vi "Frame array-Build.vi"(0 "Single-frame buffer (in)":dbl[](array[numeric]), 1 "Logging queue element":T1={"Imaging Protocol"=enum."Live Imaging", "Number of Trials"=0, "Frame Size"=512, "# Averaged frames"=0, "Dwell time (us)"=0.0, "Index of Z-plane"=0, "Timelapse?"=FALSE, "Logging process is active"=FALSE, "Speed logging enabled"=FALSE, "tdms file ref"=refnum, "path"=path "", "Trial Number"=0, "Expected # points acquired"=FALSE, "Manually stopped"=FALSE, "Last trial"=FALSE, "Ch0 data"=[], "Ch1 data"=[], "Image Time"=[], "Continuous Time"=[], "Points acquired"={"Ch0 last trial"=0, "Ch1 last trial"=0, "All trials"=0}, "HW Timings File"=refnum} {"Frame Size" items=["100X100"=100, "128X128"=128, "200X200"=200, "256X256"=256, "512X512"=512, "1024x1024"=1024, "2048x2048"=2048]; "Dwell time (us)" format="%#.6g"}, 5 "New chunk of scaled data (single channel)":dbl[](array[numeric]), 9 "Number of points in single-frame buffer (in)":i32, 11 "Frame values sum (in)":dbl[](array[numeric]), 12 "Averaged frames count (in)":i32, 13 "Number of channels in input data array":i32=1) -> (3 "Frame Data":dbl[](array[numeric]), 4 "Single-frame buffer (out)":dbl[](array[numeric]), 6 "Frame completed/generate image":bool, 10 "Number of points in single-frame buffer (out)":i32, 14 "Averaged frames count (out)":i32, 15 "Frame values sum (out)":dbl[](array[numeric]))   [LabVIEW 2017]
uses:
  Typedefs/Logging queue element.ctl
  Typedefs/Imaging Protocols enum.ctl
  Typedefs/Frame Size.ctl
  Typedefs/Acquired points count.ctl
panel:
  out "# Averaged frames":u16
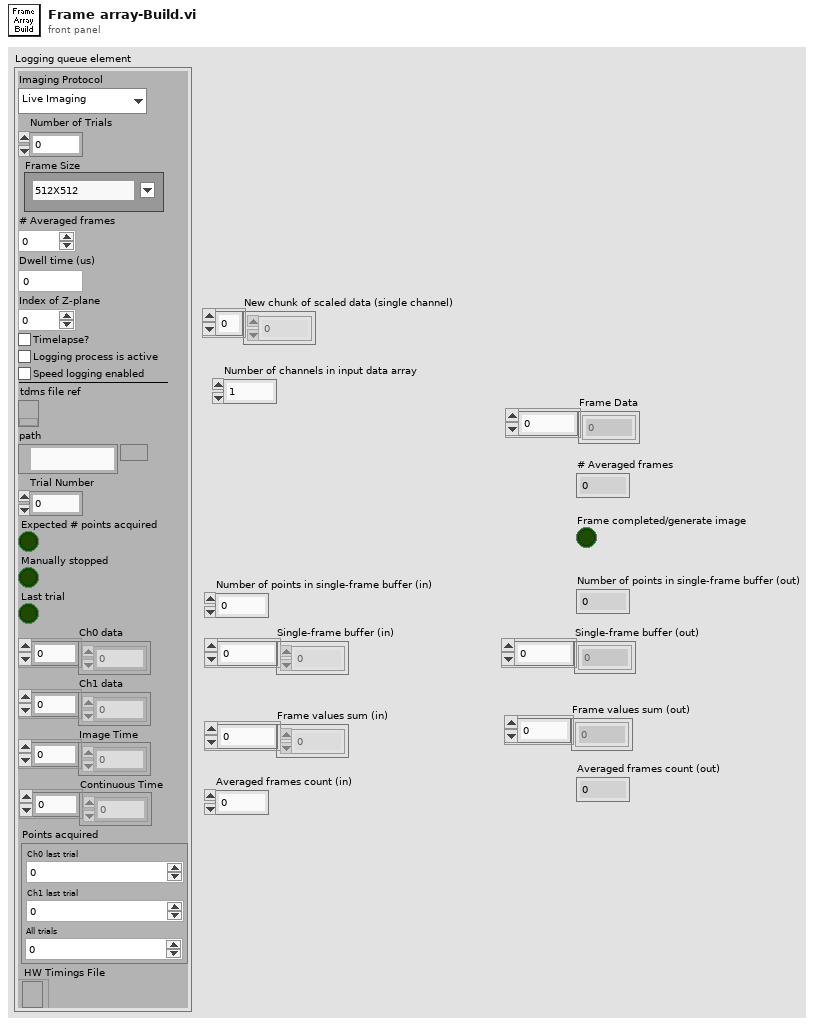
[diagram p1: front panel]
types:
  T1 = typedef "Logging queue element.ctl" = cluster{"Imaging Protocol":T2, "Number of Trials":u16, "Frame Size":T3, "# Averaged frames":u16, "Dwell time (us)":dbl, "Index of Z-plane":i32, "Timelapse?":bool, "Logging process is active":bool, "Speed logging enabled":bool, "tdms file ref":refnum<k34>, "path":path, "Trial Number":i32, "Expected # points acquired":bool, "Manually stopped":bool, "Last trial":bool, "Ch0 data":u32[], "Ch1 data":u32[], "Image Time":u64[], "Continuous Time":u64[], "Points acquired":T4, "HW Timings File":refnum<file>}
  T2 = typedef "Imaging Protocols enum.ctl" = enum16{"AOL Z-Stack", "Motor Z Stack", "Functional Acquisition", "Single Plane Acquisition", "Volume Acquisition", "Live Imaging", "Live Plane Imaging", "Live Volume Imaging"}
  T3 = typedef "Frame Size.ctl" = u16
  T4 = typedef "Acquired points count.ctl" = cluster{"Ch0 last trial":u64, "Ch1 last trial":u64, "All trials":u64}
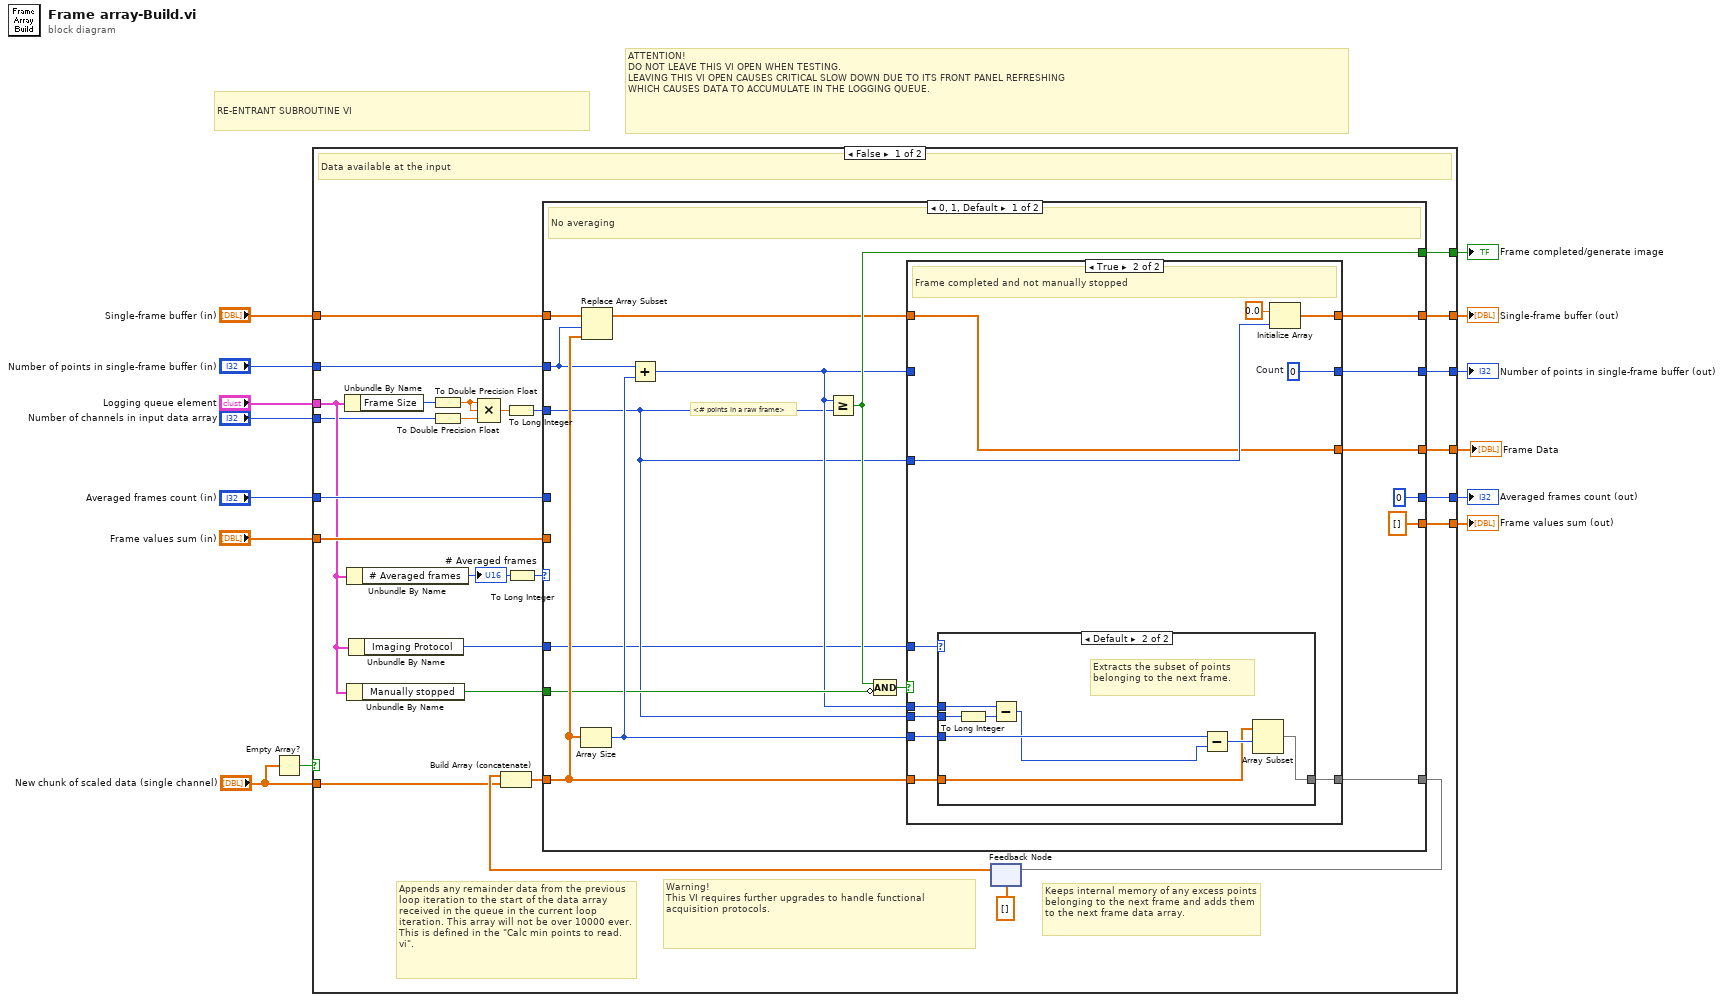
[diagram p0: block diagram]
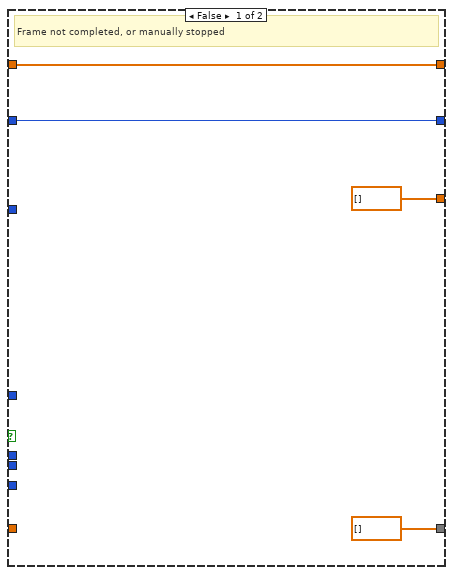
[diagram p2: hidden frame]
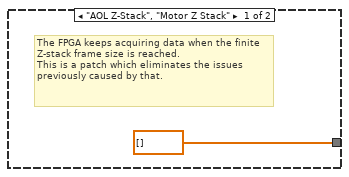
[diagram p3: hidden frame]
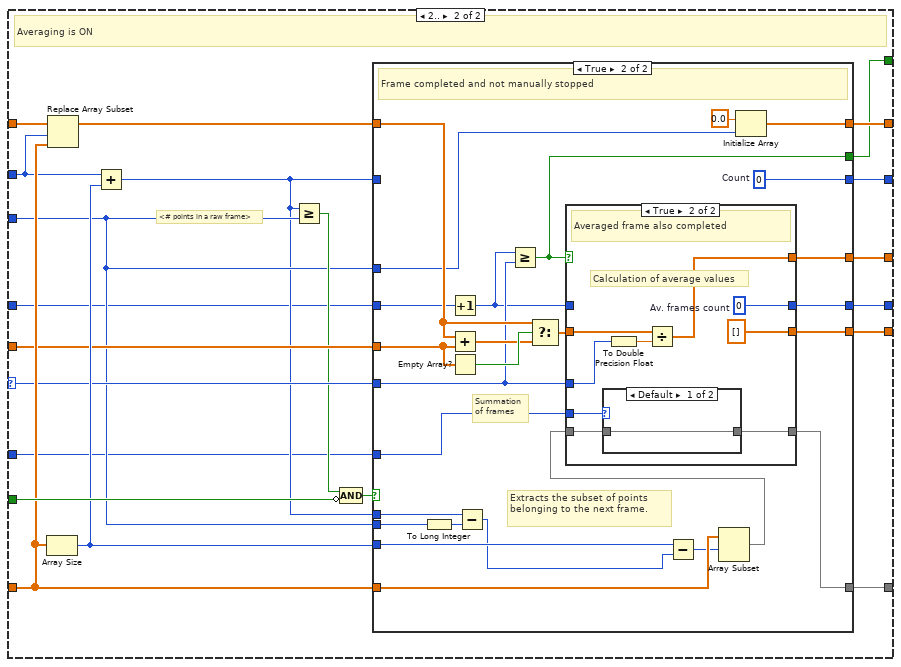
[diagram p4: hidden frame]
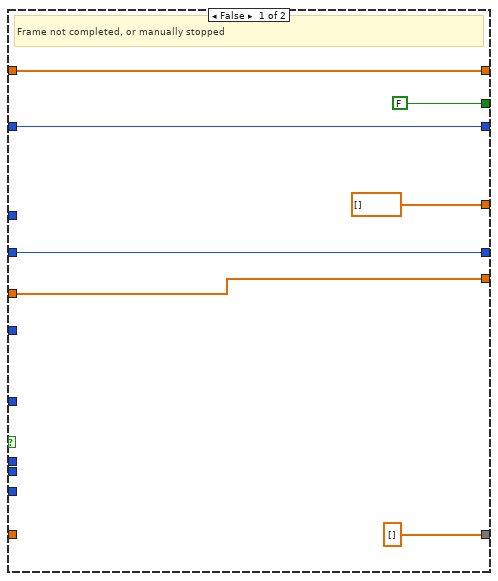
[diagram p5: hidden frame]
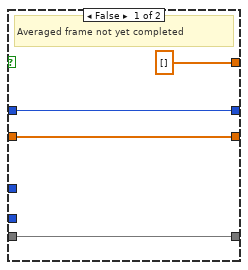
[diagram p6: hidden frame]
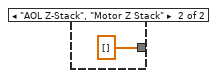
[diagram p7: hidden frame]
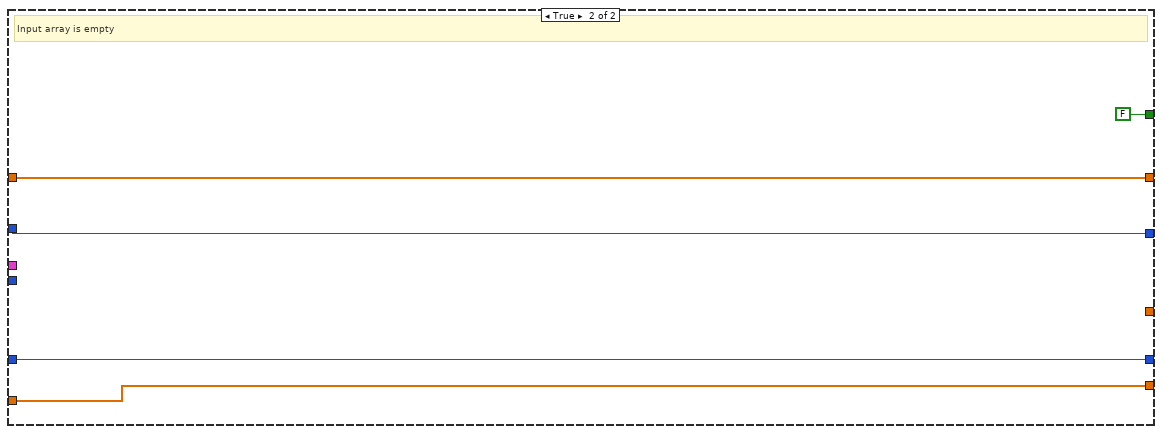
[diagram p8: hidden frame]
diagram:
  # "ATTENTION!\nDO NOT LEAVE THIS VI OPEN WHEN TESTING.\nLEAVING THIS VI OPEN CAUSES CRITICAL SLOW DOWN DUE TO ITS FRONT PANEL REFRESHING\nWHICH CAUSES DATA TO ACCUMULATE IN THE LOGGING QUEUE."
  # "RE-ENTRANT SUBROUTINE VI"
  n1 = Empty Array?(array="New chunk of scaled data (single channel)") -> (empty?=w1:bool)
  n2 = case shown="False" w1 {
    tunnel: "Number of points in single-frame buffer (in)" -> [w40 w154]
    tunnel: [w39 FALSE] -> w13
    tunnel: "Single-frame buffer (in)" -> [w38 w155]
    tunnel: [w37 w154] -> w11
    tunnel: "Frame values sum (in)" -> [w36 w151]
    tunnel: [w35 w151] -> w9
    tunnel: [w34 w155] -> w8
    tunnel: [w33 _] -> w7
    tunnel: [w32 w153] -> w6
    tunnel: "Averaged frames count (in)" -> [w31 w153]
    tunnel: "Logging queue element" -> [w20 _]
    tunnel: "New chunk of scaled data (single channel)" -> [w18 _]
    tunnel: "Number of channels in input data array" -> [w17 _]
    frame False {
      # "Warning!\nThis VI requires further upgrades to handle functional acquisition protocols."
      # "Appends any remainder data from the previous loop iteration to the start of the data array received in the queue in the current loop iteration. This array will not be over 10000 ever. This is defined in the \"Calc min points to read.vi\"."
      # "Keeps internal memory of any excess points belonging to the next frame and adds them to the next frame data array."
      # "Data available at the input"
      n3 = Unbundle By Name(w20) -> ("Frame Size"=w29:T3)
      n4 = Unbundle By Name(w20) -> ("# Averaged frames"=w24:u16)
      "# Averaged frames" <- w24
      n5 = Unbundle By Name(w20) -> ("Manually stopped"=w27:bool)
      n6 = Unbundle By Name(w20) -> ("Imaging Protocol"=w19:T2)
      n7 = To Double Precision Float(number=w29) -> (double precision float=w26:dbl)
      n8 = To Double Precision Float(number=w17) -> (double precision float=w16:dbl)
      n9 = Compound Arithmetic op=MULTIPLY(w26, w26, w16) -> (w25:dbl)
      n10 = To Long Integer(number=w25) -> (32bit integer=w15:i32)
      n11 = To Long Integer(number=w24) -> (32bit integer=w22:i32)
      n12 = feedback #1(dbl[] []) -> (w23:dbl[])
      n13 = Build Array (concatenate)(w23, w18) -> (w21:dbl[])
      n14 = case shown="0, 1, Default" w22 {
        selector: w22 -> [_ w94]
        tunnel: [w57 w102] -> w30
        tunnel: [w56 w84] -> w39
        tunnel: w27 -> [w49 w100]
        tunnel: w21 -> [w54 w99]
        tunnel: [w47 w89] -> w34
        tunnel: w38 -> [w53 w98]
        tunnel: w40 -> [w52 w97]
        tunnel: w15 -> [w45 w91]
        tunnel: [w46 w87] -> w37
        tunnel: w36 -> [_ w95]
        tunnel: [dbl[] [] ("Averaged frame values sum (in)") w92] -> w35
        tunnel: [w44 w86] -> w33
        tunnel: [0 ("Av. frames count") w85] -> w32
        tunnel: w31 -> [_ w83]
        tunnel: w19 -> [w41 w82]
        frame 0, 1, Default {
          # "<# points in a raw frame>"
          # "No averaging"
          n15 = Array Size(array=w54) -> (size(s)=w51:i32)
          n16 = Replace Array Subset "Replace Array Subset"(array=w53, new element=w54, index=w52) -> (w42:dbl[])
          n17 = Add(x=w52, y=w51) -> (x+y=w48:i32)
          n18 = Greater Or Equal?(x=w48, y=w45) -> (x >= y?=w56:bool)
          n19 = Compound Arithmetic op=AND(w56, invert w49) -> (w55:bool)
          n20 = case shown="True" w55 {
            tunnel: w48 -> [_ w72]
            tunnel: w54 -> [_ w70]
            tunnel: w51 -> [_ w71]
            tunnel: [dbl[] [] w69] -> w57
            tunnel: w45 -> [_ w68]
            tunnel: w42 -> [w59 w63]
            tunnel: w48 -> [w60 _]
            tunnel: [w60 w64] -> w46
            tunnel: [w59 w66] -> w47
            tunnel: w45 -> [_ w65]
            tunnel: [dbl[] [] w63] -> w44
            tunnel: w41 -> [_ w62]
            frame False {
              # "Frame not completed, or manually stopped"
            }
            frame True {
              w64 = 0  # Count
              # "Frame completed and not manually stopped"
              n21 = case shown="Default" w62 {
                tunnel: w72 -> [_ w81]
                tunnel: w71 -> [_ w79]
                tunnel: w70 -> [_ w76]
                tunnel: [dbl[] [] w75] -> w69
                tunnel: w68 -> [_ w74]
                frame "AOL Z-Stack", "Motor Z Stack" {
                  # "The FPGA keeps acquiring data when the finite Z-stack frame size is reached.\nThis is a patch which eliminates the issues previously caused by that."
                }
                frame Default {
                  # "Extracts the subset of points belonging to the next frame."
                  n22 = To Long Integer(number=w74) -> (32bit integer=w80:i32)
                  n23 = Subtract(x=w81, y=w80) -> (x-y=w78:i32)
                  n24 = Subtract(x=w79, y=w78) -> (x-y=w77:i32)
                  n25 = Array Subset "Array Subset"(array=w76, index=w77) -> (w75:dbl[])  [unwired: 1 in]
                }
              }
              n26 = Initialize Array(0.0, w65) -> (w66:dbl[])
            }
          }
        }
        frame 2.. {
          # "<# points in a raw frame>"
          # "Averaging is ON"
          n27 = Array Size(array=w99) -> (size(s)=w96:i32)
          n28 = Replace Array Subset "Replace Array Subset"(array=w98, new element=w99, index=w97) -> (w90:dbl[])
          n29 = Add(x=w97, y=w96) -> (x+y=w88:i32)
          n30 = Greater Or Equal?(x=w88, y=w91) -> (x >= y?=w93:bool)
          n31 = Compound Arithmetic op=AND(w93, invert w100) -> (w101:bool)
          n32 = case shown="True" w101 {
            tunnel: w88 -> [_ w135]
            tunnel: w99 -> [_ w134]
            tunnel: w96 -> [_ w116]
            tunnel: [dbl[] [] w110] -> w102
            tunnel: w91 -> [_ w133]
            tunnel: w90 -> [w107 w131]
            tunnel: w95 -> [w108 w132]
            tunnel: [w108 w119] -> w92
            tunnel: w94 -> [_ w121]
            tunnel: [w107 w126] -> w89
            tunnel: w91 -> [_ w125]
            tunnel: w88 -> [w106 _]
            tunnel: [w106 w124] -> w87
            tunnel: [dbl[] [] w123] -> w86
            tunnel: [w104 w118] -> w85
            tunnel: [FALSE w122] -> w84
            tunnel: w83 -> [w104 w120]
            tunnel: w82 -> [_ w112]
            frame False {
              # "Frame not completed, or manually stopped"
            }
            frame True {
              w124 = 0  # Count
              # "Extracts the subset of points belonging to the next frame."
              # "Summation of frames"
              # "Frame completed and not manually stopped"
              n33 = To Long Integer(number=w133) -> (32bit integer=w115:i32)
              n34 = Increment(x=w120) -> (x+1=w117:i32)
              n35 = Add(x=w131, y=w132) -> (x+y=w129:dbl[])
              n36 = Empty Array?(array=w132) -> (empty?=w130:bool)
              n37 = Subtract(x=w135, y=w115) -> (x-y=w114:i32)
              n38 = Greater Or Equal?(x=w117, y=w121) -> (x >= y?=w122:bool)
              n39 = Select(t=w131, s=w130, f=w129) -> (s? t:f=w128:dbl[])
              n40 = Subtract(x=w116, y=w114) -> (x-y=w113:i32)
              n41 = Array Subset "Array Subset"(array=w134, index=w113) -> (w111:dbl[])  [unwired: 1 in]
              n42 = case shown="True" w122 {
                tunnel: [dbl[] [] ("Frame-size data array out") w145] -> w123
                tunnel: w121 -> [_ w147]
                tunnel: w128 -> [w139 w148]
                tunnel: [w139 dbl[] [] ("Frame-size data array out")] -> w119
                tunnel: w117 -> [w137 _]
                tunnel: [w137 w143] -> w118
                tunnel: w111 -> [w136 w141]
                tunnel: w112 -> [_ w142]
                tunnel: [w136 w140] -> w110
                frame False {
                  # "Averaged frame not yet completed"
                }
                frame True {
                  w143 = 0  # Av. frames count
                  # "Calculation of average values"
                  # "Averaged frame also completed"
                  n43 = case shown="Default" w142 {
                    tunnel: w141 -> [w149 _]
                    tunnel: [w149 dbl[] [] ("Frame-size data array out")] -> w140
                    frame Default {
                    }
                    frame "AOL Z-Stack", "Motor Z Stack" {
                    }
                  }
                  n44 = To Double Precision Float(number=w147) -> (double precision float=w146:dbl)
                  n45 = Divide(x=w148, y=w146) -> (x/y=w145:dbl[])
                }
              }
              n46 = Initialize Array(0.0, w125) -> (w126:dbl[])
            }
          }
        }
      }
      n47 = feedback-in #1(w30) -> ()
    }
    frame True {
      # "Input array is empty"
    }
  }
  "Number of points in single-frame buffer (out)" <- w11
  "Single-frame buffer (out)" <- w8
  "Frame completed/generate image" <- w13
  "Frame values sum (out)" <- w9
  "Frame Data" <- w7
  "Averaged frames count (out)" <- w6
